vi "Benchmark Massdata.vi"() -> ()   [LabVIEW 2020]
uses:
  185e4978-8efa-4451-b18b-c5c5d5291fa2.vi
  95340353-4e09-47c7-b912-a3c63f0b7fd3.vi
  <userlib>/_NEVSTOP/Communicable State Machine(CSM)/addons/MassData-Parameter/_support/FGV-MassData.vi
  <userlib>/_NEVSTOP/Communicable State Machine(CSM)/Communicable State Machine.lvlib
panel:
  out "inside 3":i32
  out "outside 3":i32
  out "ratio":dbl[](graph)
  out "inside 2":i32
  out "outside 2":i32
  out "inside":i32
  out "outside":i32
  out "unit (ms)":dbl[][](graph)
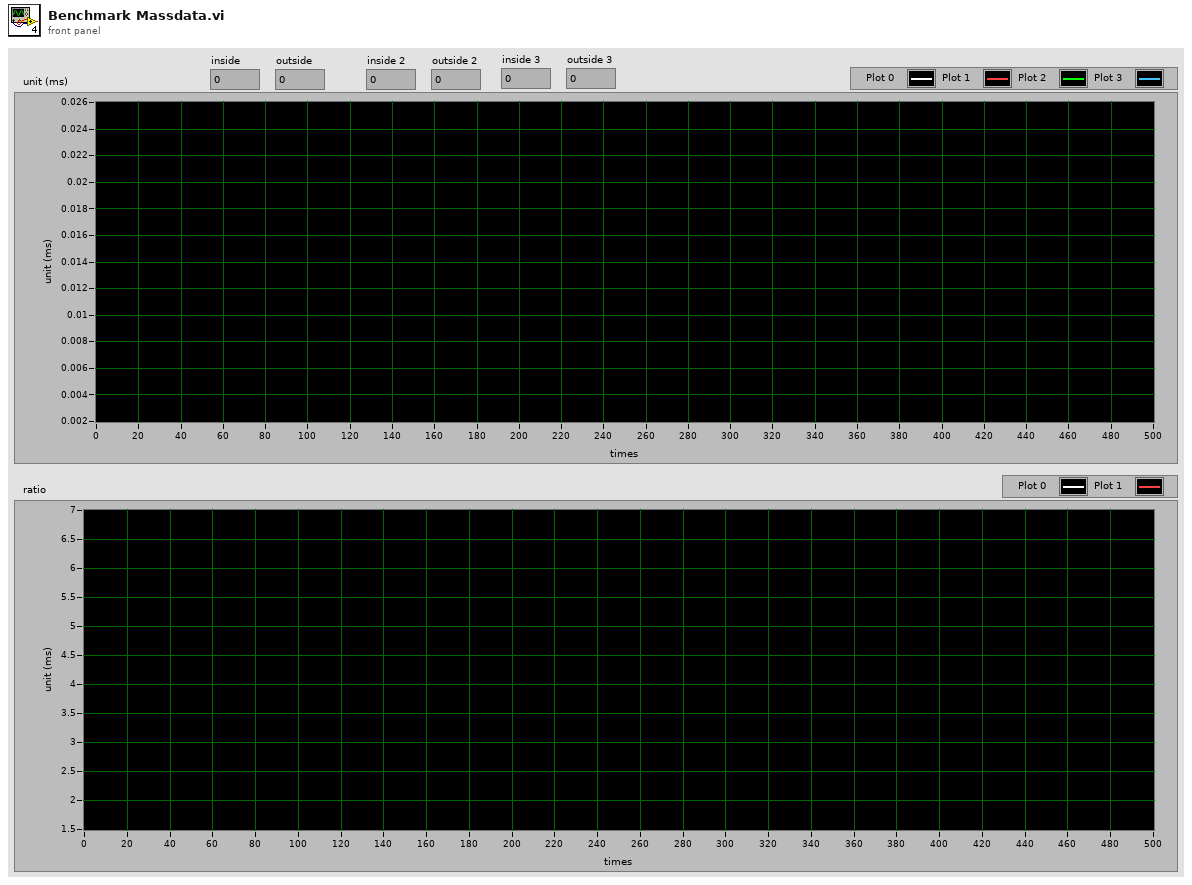
[diagram p1: front panel]
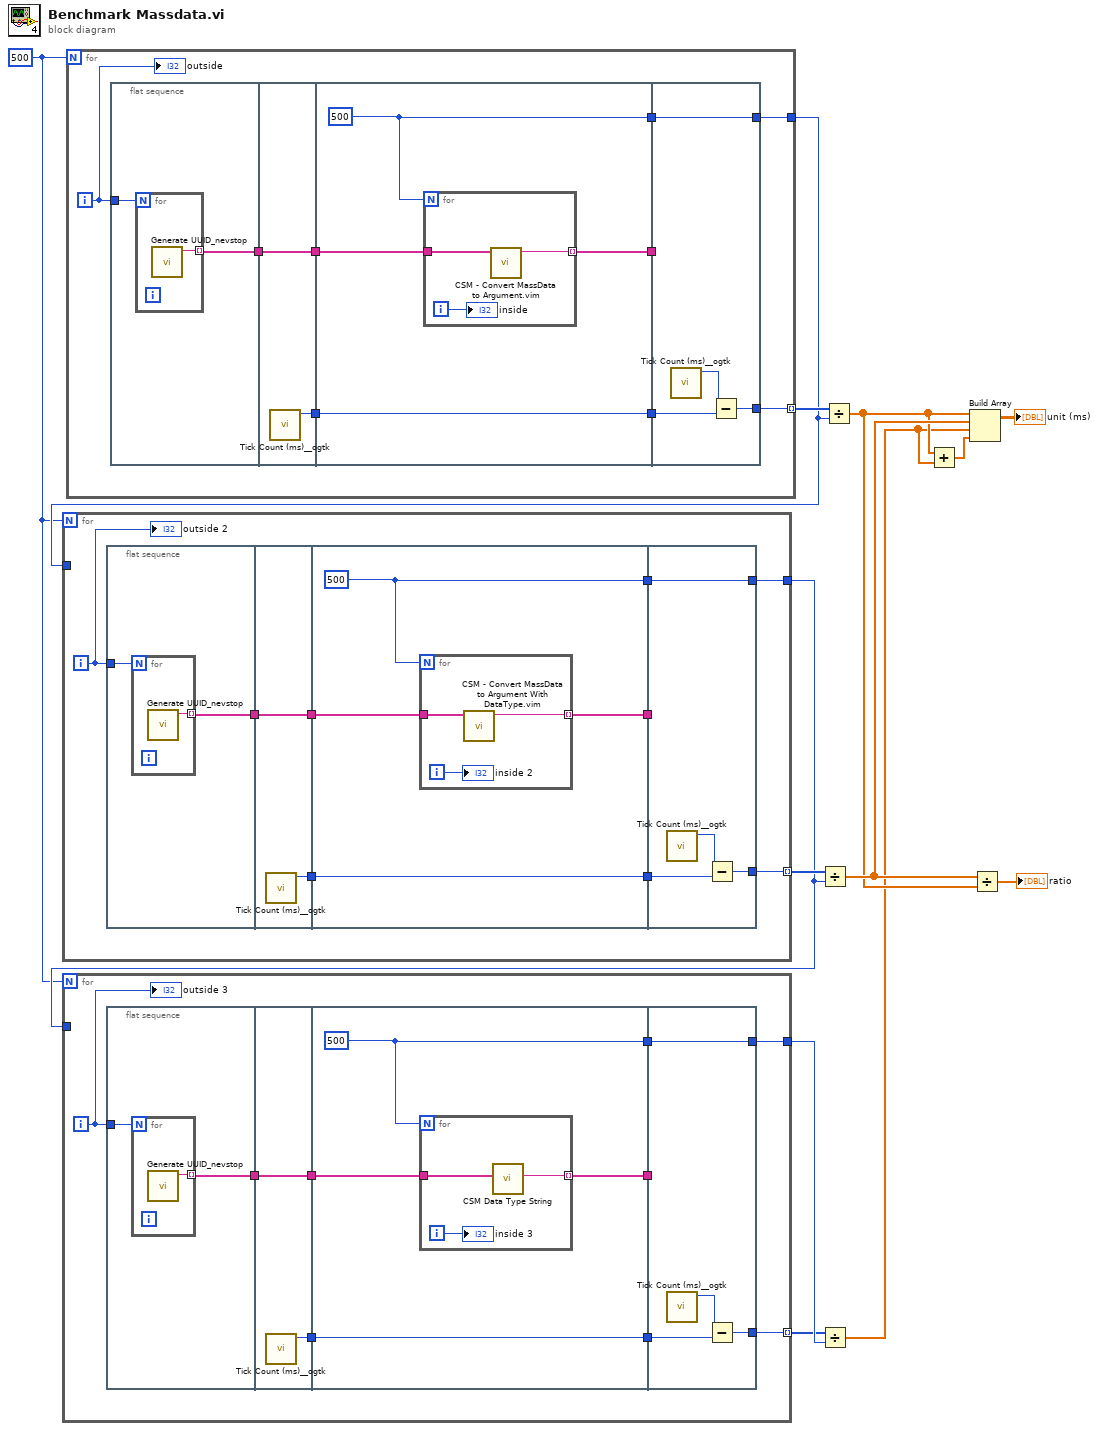
[diagram p0: block diagram]
diagram:
  w1 = 500
  n1 = for {
    N: w1 -> [_]
    tunnel: [w20] -> w13 mode=indexing
    tunnel: [w19] -> w11
    i -> [w17]
    n2 = flat-sequence {
      tunnel: w17 -> [w24]
      tunnel: [w23] -> w16
      tunnel: [w27] -> w22
      tunnel: w16 -> [w26]
      tunnel: [w26] -> w15
      tunnel: w22 -> [w31]
      tunnel: [w31] -> w21
      tunnel: [w30] -> w18
      tunnel: w15 -> [w29]
      tunnel: [w28] -> w14
      tunnel: w21 -> [w37]
      tunnel: [w36] -> w20
      tunnel: [w35] -> w19
      tunnel: w18 -> [w35]
      tunnel: w14 -> [_]
      frame #0 {
        n3 = for {
          N: w24 -> [_]
          tunnel: [w25] -> w23 mode=indexing
          n4 = call <userlib>:"Generate UUID_nevstop.vi"() -> ("UUID"=w25:string)  [unwired: 11 in]
        }
      }
      frame #1 {
        n5 = call <userlib>:"Tick Count (ms)__ogtk.vi"() -> ("millisecond timer value"=w27:u32)  [unwired: 10 in, 1 out]
      }
      frame #2 {
        w30 = 500
        n6 = for {
          N: w30 -> [_]
          tunnel: w29 -> [w33]
          tunnel: [w32] -> w28 mode=indexing
          i -> [w34]
          n7 = call "CSM - Convert MassData to Argument.vim"("DBL"=w33) -> ("MassData Argument"=w32:string)  [unwired: 7 in, 1 out]
          "inside" <- w34
        }
      }
      frame #3 {
        n8 = call <userlib>:"Tick Count (ms)__ogtk.vi"() -> ("millisecond timer value"=w38:u32)  [unwired: 10 in, 1 out]
        n9 = Subtract(x=w38, y=w37) -> (x-y=w36:u32)
      }
    }
    "outside" <- w17
  }
  n10 = for {
    N: w1 -> [_]
    tunnel: [w45] -> w12 mode=indexing
    tunnel: [w44] -> w5
    tunnel: w11 -> [_]
    i -> [w42]
    n11 = flat-sequence {
      tunnel: w42 -> [w49]
      tunnel: [w48] -> w41
      tunnel: [w52] -> w47
      tunnel: w41 -> [w51]
      tunnel: [w51] -> w40
      tunnel: w47 -> [w56]
      tunnel: [w56] -> w46
      tunnel: [w55] -> w43
      tunnel: w40 -> [w54]
      tunnel: [w53] -> w39
      tunnel: w46 -> [w62]
      tunnel: [w61] -> w45
      tunnel: [w60] -> w44
      tunnel: w43 -> [w60]
      tunnel: w39 -> [_]
      frame #0 {
        n12 = for {
          N: w49 -> [_]
          tunnel: [w50] -> w48 mode=indexing
          n13 = call <userlib>:"Generate UUID_nevstop.vi"() -> ("UUID"=w50:string)  [unwired: 11 in]
        }
      }
      frame #1 {
        n14 = call <userlib>:"Tick Count (ms)__ogtk.vi"() -> ("millisecond timer value"=w52:u32)  [unwired: 10 in, 1 out]
      }
      frame #2 {
        w55 = 500
        n15 = for {
          N: w55 -> [_]
          tunnel: w54 -> [w58]
          tunnel: [w57] -> w53 mode=indexing
          i -> [w59]
          n16 = call "CSM - Convert MassData to Argument With DataType.vim"("DBL"=w58) -> ("Argument"=w57:string)  [unwired: 7 in, 1 out]
          "inside 2" <- w59
        }
      }
      frame #3 {
        n17 = call <userlib>:"Tick Count (ms)__ogtk.vi"() -> ("millisecond timer value"=w63:u32)  [unwired: 10 in, 1 out]
        n18 = Subtract(x=w63, y=w62) -> (x-y=w61:u32)
      }
    }
    "outside 2" <- w42
  }
  n19 = for {
    N: w1 -> [_]
    tunnel: [w70] -> w6 mode=indexing
    tunnel: [w69] -> w7
    tunnel: w5 -> [_]
    i -> [w67]
    n20 = flat-sequence {
      tunnel: w67 -> [w74]
      tunnel: [w73] -> w66
      tunnel: [w77] -> w72
      tunnel: w66 -> [w76]
      tunnel: [w76] -> w65
      tunnel: w72 -> [w81]
      tunnel: [w81] -> w71
      tunnel: [w80] -> w68
      tunnel: w65 -> [w79]
      tunnel: [w78] -> w64
      tunnel: w71 -> [w87]
      tunnel: [w86] -> w70
      tunnel: [w85] -> w69
      tunnel: w68 -> [w85]
      tunnel: w64 -> [_]
      frame #0 {
        n21 = for {
          N: w74 -> [_]
          tunnel: [w75] -> w73 mode=indexing
          n22 = call <userlib>:"Generate UUID_nevstop.vi"() -> ("UUID"=w75:string)  [unwired: 11 in]
        }
      }
      frame #1 {
        n23 = call <userlib>:"Tick Count (ms)__ogtk.vi"() -> ("millisecond timer value"=w77:u32)  [unwired: 10 in, 1 out]
      }
      frame #2 {
        w80 = 500
        n24 = for {
          N: w80 -> [_]
          tunnel: w79 -> [w83]
          tunnel: [w82] -> w78 mode=indexing
          i -> [w84]
          n25 = call <userlib>:"CSM Data Type String.vi"("Data"=w83) -> ("Data Type String"=w82:string)  [unwired: 10 in]
          "inside 3" <- w84
        }
      }
      frame #3 {
        n26 = call <userlib>:"Tick Count (ms)__ogtk.vi"() -> ("millisecond timer value"=w88:u32)  [unwired: 10 in, 1 out]
        n27 = Subtract(x=w88, y=w87) -> (x-y=w86:u32)
      }
    }
    "outside 3" <- w67
  }
  n28 = Divide(x=w12, y=w5) -> (x/y=w9:dbl[])
  n29 = Divide(x=w6, y=w7) -> (x/y=w3:dbl[])
  n30 = Divide(x=w13, y=w11) -> (x/y=w4:dbl[])
  n31 = Add(x=w4, y=w3) -> (x+y=w2:dbl[])
  n32 = Build Array(w4, w9, w3, w2) -> (→"unit (ms)":dbl[][])
  n33 = Divide(x=w9, y=w4) -> (x/y=→"ratio":dbl[])
